vi "GlobalRegistry.vi"() -> ()   [LabVIEW 2010]
panel:
  out "Registry":T1(array[cluster])
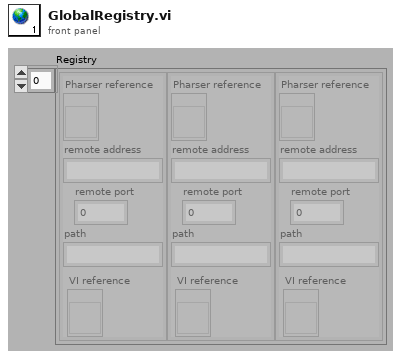
[diagram p1: front panel]
types:
  T1 = cluster{"Pharser reference":refnum<vi>, "remote address":string, "remote port":u16, "path":string, "VI reference":refnum<vi>}[]
diagram:
